vi "m1m3_getNextSample_HardpointStatus.vi"(8 "error in (no error)":errorcluster, 11 "HardpointStatus_Ctl":T1={"Timestamp"=0.0, "Mode[6]"=[0, 0, 0, 0, 0, 0], "MajorFault[6]"=[FALSE, FALSE, FALSE, FALSE, FALSE, FALSE], "MinorFault[6]"=[FALSE, FALSE, FALSE, FALSE, FALSE, FALSE], "FaultOverridden[6]"=[FALSE, FALSE, FALSE, FALSE, FALSE, FALSE], "WatchdogReset[6]"=[FALSE, FALSE, FALSE, FALSE, FALSE, FALSE], "BrownoutDetected[6]"=[FALSE, FALSE, FALSE, FALSE, FALSE, FALSE], "EventTrapReset[6]"=[FALSE, FALSE, FALSE, FALSE, FALSE, FALSE], "MotorPowerFault[6]"=[FALSE, FALSE, FALSE, FALSE, FALSE, FALSE], "SSRPowerFault[6]"=[FALSE, FALSE, FALSE, FALSE, FALSE, FALSE], "AUXPowerFault[6]"=[FALSE, FALSE, FALSE, FALSE, FALSE, FALSE], "SMCPowerFault[6]"=[FALSE, FALSE, FALSE, FALSE, FALSE, FALSE]}) -> (0 "error out":errorcluster, 2 "function return":i32, 3 "HardpointStatus_Ctl out":T1)   [LabVIEW 2016, in "SALLV_m1m3.lvlib"]
doc: "int m1m3_shm_getNextSample_HardpointStatusLV(m1m3_HardpointStatusLV *HardpointStatus_Ctl );"
uses:
  SALLV_m1m3.lvlib
  DataTypes/HardpointStatus.ctl
  SALLV_m1m3.so
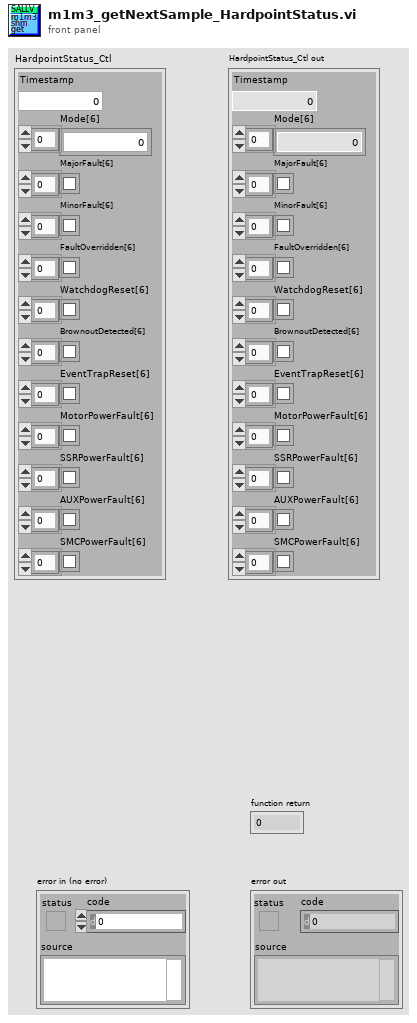
[diagram p1: front panel]
types:
  T1 = typedef "SALLV_m1m3.lvlib/HardpointStatus.ctl" = cluster{"Timestamp":dbl, "Mode[6]":u8[], "MajorFault[6]":bool[], "MinorFault[6]":bool[], "FaultOverridden[6]":bool[], "WatchdogReset[6]":bool[], "BrownoutDetected[6]":bool[], "EventTrapReset[6]":bool[], "MotorPowerFault[6]":bool[], "SSRPowerFault[6]":bool[], "AUXPowerFault[6]":bool[], "SMCPowerFault[6]":bool[]}
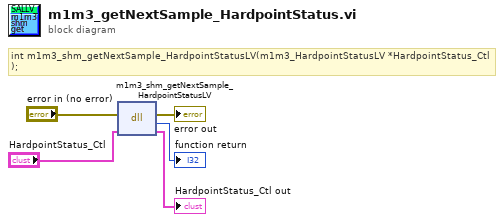
[diagram p0: block diagram]
diagram:
  # "int m1m3_shm_getNextSample_HardpointStatusLV(m1m3_HardpointStatusLV *HardpointStatus_Ctl );"
  n1 = dll-call lib="opt/CODE/SALLV_m1m3/SALLV_m1m3.*" fn="m1m3_shm_getNextSample_HardpointStatusLV"(error in="error in (no error)", "HardpointStatus_Ctl"="HardpointStatus_Ctl") -> (error out=→"error out":errorcluster, →"function return":i32, "HardpointStatus_Ctl"=→"HardpointStatus_Ctl out":T1)  [unwired: 2 in, 1 out]
